vi "Associated Power Technologies 8500 Series Manual Mode.vi"() -> ()   [LabVIEW 2014]
doc: "This VI is an example for controlling the power source, APT-8500 series, of Associated Power Technologies. \n\nThe manual mode is a fundamental function to output a configured voltage ."
uses:
  <instrlib>/Associated Power Technologies 8500 Series/Public/Configure/Manual Mode/Manual Mode - Add File.vi
  <instrlib>/Associated Power Technologies 8500 Series/Public/Configure/Manual Mode/Manual Mode - Edit File.vi
  <instrlib>/Associated Power Technologies 8500 Series/Public/Configure/Manual Mode/Manual Mode - Configure Output Couple.vi
  <instrlib>/Associated Power Technologies 8500 Series/Public/Configure/Manual Mode/Manual Mode - Configure Range.vi
  <instrlib>/Associated Power Technologies 8500 Series/Public/Configure/Manual Mode/Manual Mode - Configure Output Waveform.vi
  <instrlib>/Associated Power Technologies 8500 Series/Public/Configure/Manual Mode/Manual Mode - Configure AC Voltage.vi
  <instrlib>/Associated Power Technologies 8500 Series/Public/Configure/Manual Mode/Manual Mode - Configure Frequency.vi
  <instrlib>/Associated Power Technologies 8500 Series/Public/Configure/Manual Mode/Manual Mode - Configure Start Angle.vi
  <instrlib>/Associated Power Technologies 8500 Series/Public/Configure/Manual Mode/Manual Mode - Configure DC Voltage.vi
  <instrlib>/Associated Power Technologies 8500 Series/Public/Configure/Manual Mode/Manual Mode - Configure Ramp up time.vi
  <instrlib>/Associated Power Technologies 8500 Series/Public/Configure/Manual Mode/Manual Mode - Configure High Limitation of Current.vi
  <instrlib>/Associated Power Technologies 8500 Series/Public/Configure/Manual Mode/Manual Mode - Configure High Limitation of Power.vi
  <instrlib>/Associated Power Technologies 8500 Series/Public/Configure/Manual Mode/Manual Mode - Configure Delay Time of High Limitation.vi
  <instrlib>/Associated Power Technologies 8500 Series/Public/Configure/Manual Mode/Manual Mode - Configure THD.vi
  <instrlib>/Associated Power Technologies 8500 Series/Public/Configure/Manual Mode/Manual Mode - Load File.vi
  <instrlib>/Associated Power Technologies 8500 Series/Public/Data/Measurement/Read All Measurements.vi
  <instrlib>/Associated Power Technologies 8500 Series/Associated Power Technologies 8500 Series.lvlib
panel:
  out "All Measurements":T1
  in  "File Name":string="EXAMPLE"
  in  "Stop":bool
  in  "Manual Mode Parameters":T2={"Couple"=2, "Waveform Type"=0, "Range"=0, "AC Voltage"=100.0, "DC Voltage"=0.0, "Frequency"=60.0, "Ramp Up Time(s)"=0.0, "Start Angle(degree)"=0, "A-HI(A)"=0.0, "P-HI(W)"=0, "Delay(s)"=0.0, "THD"=0.0} {"THD" min=0.0 max=46.0 step=0.1; "Couple" items=["AC", "DC", "ACDC"]; "Waveform Type" items=["Sine", "Triangle", "Square", "Clipped"]; "Range" items=["AUTO", "HIGH", "LOW"]; "AC Voltage" min=0.0 max=310.0; "DC Voltage" min=0.0 max=420.0; "Frequency" min=5.0 max=1200.0; "Ramp Up Time(s)" min=0.0 max=999.9 step=0.1; "Start Angle(degree)" max=359; "A-HI(A)" min=0.0; "Delay(s)" min=0.0 max=999.9 step=0.1}
  in  "Serial Configuration":T3={"Baud Rate"=115200, "Parity"=0, "Data Bits"=8, "Stop Bits"=10, "Flow Control"=0} {"Flow Control" items=["None", "XON/XOFF", "RTS/CTS", "XON/XOFF & RTS/CTS", "DTR/DSR", "XON/XOFF & DTR/DSR"]; "Stop Bits" items=["1.0"=10, "1.5"=15, "2.0"=20]; "Data Bits" items=["7"=7, "8"=8]; "Parity" items=["None", "Odd", "Even", "Mark", "Space"]; "Baud Rate" items=["300"=300, "600"=600, "1200"=1200, "2400"=2400, "4800"=4800, "9600"=9600, "19200"=19200, "38400"=38400, "115200"=115200]}
  in  "VISA resource name":refnum<visa-resource-name>
  # "Manual Mode Operation of APT-8500 Series"
  # "Initialization"
  # "Configurations"
  # "Meters"
  # "(c) 2020 Associated Power Technologies.  ALL RIGHTS RESERVED."
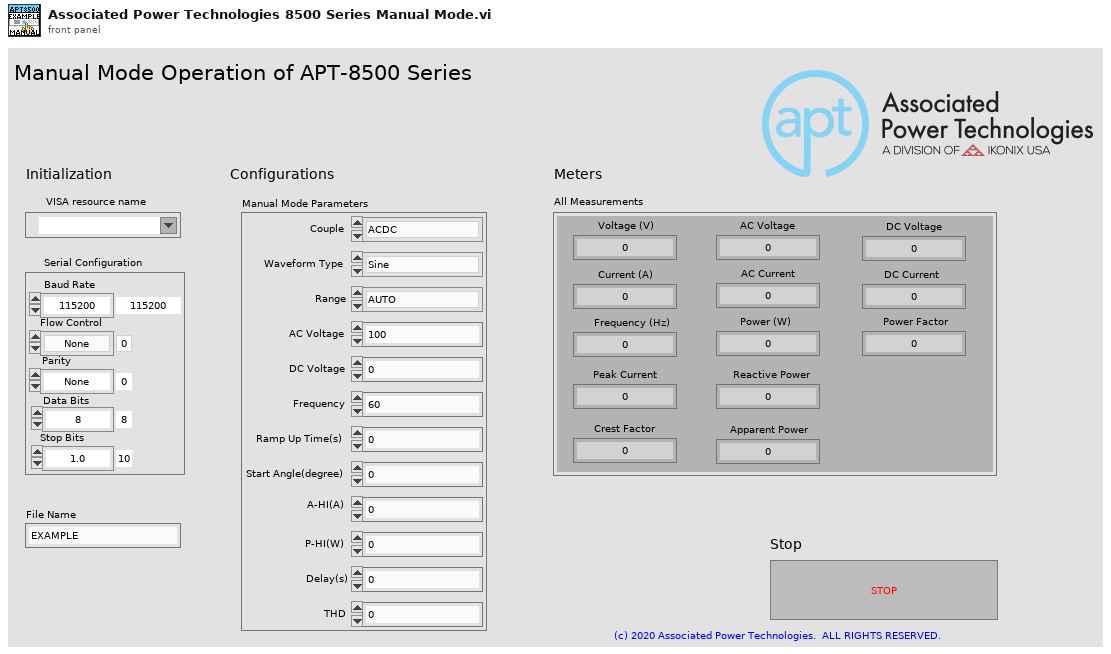
[diagram p1: front panel]
types:
  T1 = cluster{"Voltage (V)":dbl, "AC Voltage":dbl, "DC Voltage":dbl, "Current (A)":dbl, "AC Current":dbl, "DC Current":dbl, "Frequency (Hz)":dbl, "Power (W)":dbl, "Power Factor":dbl, "Peak Current":dbl, "Reactive Power":dbl, "Crest Factor":dbl, "Apparent Power":dbl}
  T2 = cluster{"Couple":u16, "Waveform Type":u16, "Range":u16, "AC Voltage":dbl, "DC Voltage":dbl, "Frequency":dbl, "Ramp Up Time(s)":dbl, "Start Angle(degree)":u16, "A-HI(A)":dbl, "P-HI(W)":u32, "Delay(s)":dbl, "THD":dbl}
  T3 = cluster{"Baud Rate":u32, "Parity":u16, "Data Bits":u16, "Stop Bits":u16, "Flow Control":u16}
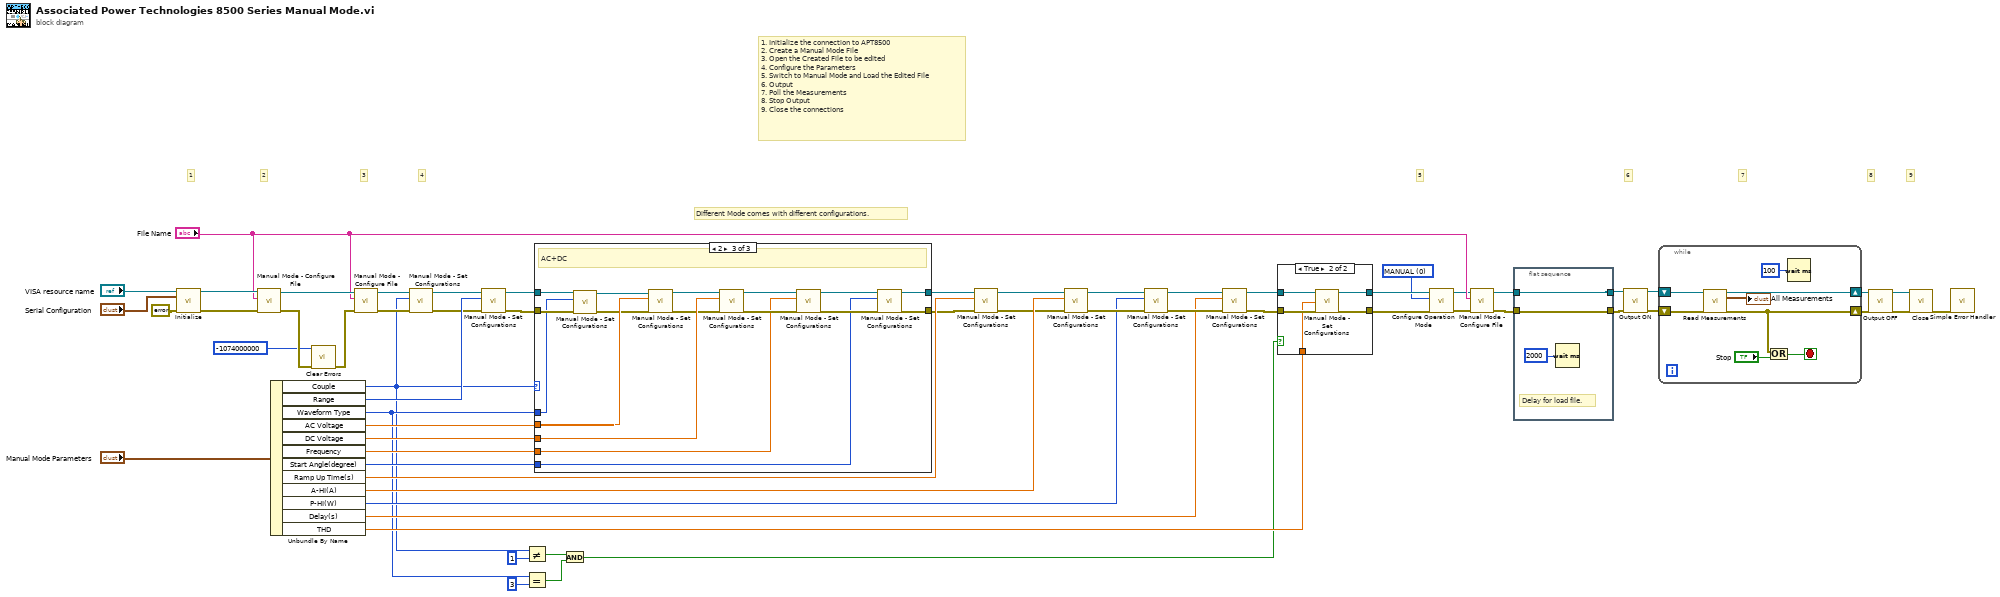
[diagram p0: block diagram]
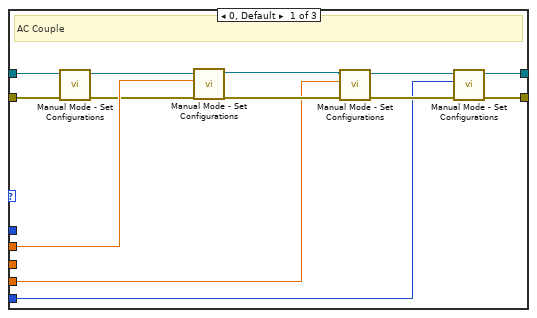
[diagram p3: hidden frame]
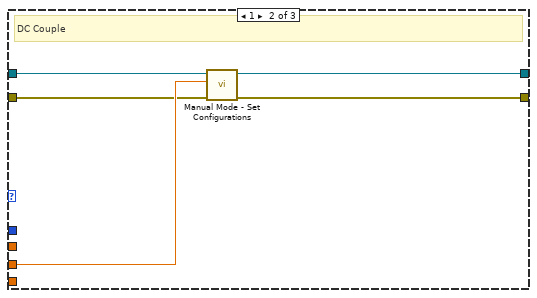
[diagram p4: hidden frame]
diagram:
  w3 = u16 0 items=["MANUAL", "LIST", "PULSE", "STEP"] ("Operation Mode")
  # "Different Mode comes with different configurations."
  # "1. Initialize the connection to APT8500\n2. Create a Manual Mode File\n3. Open the Created File to be edited\n4. Configure the Parameters\n5. Switch to Manual Mode and Load the Edited File\n6. Output\n7. Poll the Measurements\n8. Stop Output\n9. Close the connections"
  # "9"
  # "8"
  # "7"
  # "6"
  # "5"
  # "4"
  # "3"
  # "2"
  # "1"
  n1 = call <instrlib>:"Initialize.vi"("VISA resource name"="VISA resource name", "Serial Configuration"="Serial Configuration", "error in (no error)"=errorcluster {"status"=FALSE, "code"=0, "source"=""}) -> ("VISA resource name out"=w56:refnum<visa-resource-name>, "error out"=w57:errorcluster)  [unwired: 11 in]
  n2 = call-poly <instrlib>:"Manual Mode - Configure File.vi"("error in (no error)"=w57, "File Name"="File Name", "VISA resource name"=w56) -> ("error out"=w11:errorcluster, "VISA resource name out"=w55:refnum<visa-resource-name>)  [unwired: 7 in]
  n3 = Unbundle By Name("Manual Mode Parameters") -> ("Couple"=w26:u16, "Range"=w29:u16, "Waveform Type"=w28:u16, "AC Voltage"=w50:dbl, "DC Voltage"=w47:dbl, "Frequency"=w36:dbl, "Start Angle(degree)"=w32:u16, "Ramp Up Time(s)"=w33:dbl, "A-HI(A)"=w46:dbl, "P-HI(W)"=w43:u32, "Delay(s)"=w40:dbl, "THD"=w37:dbl)
  n4 = call <vilib>:"Clear Errors.vi"("error in (no error)"=w11, "specific error code to clear (0: all)"=-1074000000) -> ("error out"=w10:errorcluster)  [unwired: 4 in, 1 out]
  n5 = call-poly <instrlib>:"Manual Mode - Configure File.vi"("error in (no error)"=w10, "File Name"="File Name", "VISA resource name"=w55) -> ("error out"=w53:errorcluster, "VISA resource name out"=w54:refnum<visa-resource-name>)  [unwired: 7 in]
  n6 = call-poly <instrlib>:"Manual Mode - Set Configurations.vi"("error in (no error)"=w53, "Couple (AC)"=w26, "VISA resource name"=w54) -> ("error out"=w1:errorcluster, "VISA resource name out"=w2:refnum<visa-resource-name>)  [unwired: 7 in]
  n7 = call-poly <instrlib>:"Manual Mode - Set Configurations.vi"("error in (no error)"=w1, "Range (Auto)"=w29, "VISA resource name"=w2) -> ("error out"=w48:errorcluster, "VISA resource name out"=w49:refnum<visa-resource-name>)  [unwired: 7 in]
  n8 = Not Equal?(x=w26, y=u16 1) -> (x != y?=w23:bool)
  n9 = Equal?(x=w28, y=u16 3 ("x")) -> (x = y?=w24:bool)
  n10 = case shown="2" w26 {
    tunnel: w50 -> [w73 _ w95]
    tunnel: w49 -> [w64 w75 w83]
    tunnel: w48 -> [w62 w74 w81]
    tunnel: w47 -> [_ w78 w94]
    tunnel: [w66 w77 w86] -> w31
    tunnel: [w67 w76 w85] -> w30
    tunnel: w36 -> [w70 _ w89]
    tunnel: w32 -> [w65 _ w84]
    tunnel: w28 -> [_ _ w79]
    frame 0, Default {
      # "AC Couple"
      n11 = call-poly <instrlib>:"Manual Mode - Set Configurations.vi"("error in (no error)"=w62, "VISA resource name"=w64) -> ("error out"=w61:errorcluster, "VISA resource name out"=w63:refnum<visa-resource-name>)  [unwired: 8 in]
      n12 = call-poly <instrlib>:"Manual Mode - Set Configurations.vi"("error in (no error)"=w61, "AC Voltage (0)"=w73, "VISA resource name"=w63) -> ("error out"=w71:errorcluster, "VISA resource name out"=w72:refnum<visa-resource-name>)  [unwired: 7 in]
      n13 = call-poly <instrlib>:"Manual Mode - Set Configurations.vi"("error in (no error)"=w71, "Frequency (60)"=w70, "VISA resource name"=w72) -> ("error out"=w68:errorcluster, "VISA resource name out"=w69:refnum<visa-resource-name>)  [unwired: 7 in]
      n14 = call-poly <instrlib>:"Manual Mode - Set Configurations.vi"("error in (no error)"=w68, "Start Angle (0)"=w65, "VISA resource name"=w69) -> ("error out"=w67:errorcluster, "VISA resource name out"=w66:refnum<visa-resource-name>)  [unwired: 7 in]
    }
    frame 1 {
      # "DC Couple"
      n15 = call-poly <instrlib>:"Manual Mode - Set Configurations.vi"("error in (no error)"=w74, "DC Voltage (0)"=w78, "VISA resource name"=w75) -> ("error out"=w76:errorcluster, "VISA resource name out"=w77:refnum<visa-resource-name>)  [unwired: 7 in]
    }
    frame 2 {
      # "AC+DC"
      n16 = call-poly <instrlib>:"Manual Mode - Set Configurations.vi"("error in (no error)"=w81, "Waveform Type (Sine)"=w79, "VISA resource name"=w83) -> ("error out"=w80:errorcluster, "VISA resource name out"=w82:refnum<visa-resource-name>)  [unwired: 7 in]
      n17 = call-poly <instrlib>:"Manual Mode - Set Configurations.vi"("error in (no error)"=w80, "AC Voltage (0)"=w95, "VISA resource name"=w82) -> ("error out"=w92:errorcluster, "VISA resource name out"=w93:refnum<visa-resource-name>)  [unwired: 7 in]
      n18 = call-poly <instrlib>:"Manual Mode - Set Configurations.vi"("error in (no error)"=w92, "DC Voltage (0)"=w94, "VISA resource name"=w93) -> ("error out"=w91:errorcluster, "VISA resource name out"=w90:refnum<visa-resource-name>)  [unwired: 7 in]
      n19 = call-poly <instrlib>:"Manual Mode - Set Configurations.vi"("error in (no error)"=w91, "Frequency (60)"=w89, "VISA resource name"=w90) -> ("error out"=w88:errorcluster, "VISA resource name out"=w87:refnum<visa-resource-name>)  [unwired: 7 in]
      n20 = call-poly <instrlib>:"Manual Mode - Set Configurations.vi"("error in (no error)"=w88, "Start Angle (0)"=w84, "VISA resource name"=w87) -> ("error out"=w85:errorcluster, "VISA resource name out"=w86:refnum<visa-resource-name>)  [unwired: 7 in]
    }
  }
  n21 = And(x=w23, y=w24) -> (x .and. y?=w22:bool)
  n22 = call-poly <instrlib>:"Manual Mode - Set Configurations.vi"("error in (no error)"=w30, "Ramp Up Time (0)"=w33, "VISA resource name"=w31) -> ("error out"=w34:errorcluster, "VISA resource name out"=w35:refnum<visa-resource-name>)  [unwired: 7 in]
  n23 = call-poly <instrlib>:"Manual Mode - Set Configurations.vi"("error in (no error)"=w34, "A-HI(0)"=w46, "VISA resource name"=w35) -> ("error out"=w44:errorcluster, "VISA resource name out"=w45:refnum<visa-resource-name>)  [unwired: 7 in]
  n24 = call-poly <instrlib>:"Manual Mode - Set Configurations.vi"("error in (no error)"=w44, "P-HI(0)"=w43, "VISA resource name"=w45) -> ("error out"=w41:errorcluster, "VISA resource name out"=w42:refnum<visa-resource-name>)  [unwired: 7 in]
  n25 = call-poly <instrlib>:"Manual Mode - Set Configurations.vi"("error in (no error)"=w41, "Delay(0)"=w40, "VISA resource name"=w42) -> ("error out"=w38:errorcluster, "VISA resource name out"=w39:refnum<visa-resource-name>)  [unwired: 7 in]
  n26 = case shown="True" w22 {
    tunnel: w39 -> [w97 w102]
    tunnel: w38 -> [w96 w101]
    tunnel: w37 -> [_ w100]
    tunnel: [w97 w99] -> w6
    tunnel: [w96 w98] -> w5
    frame False {
    }
    frame True {
      n27 = call-poly <instrlib>:"Manual Mode - Set Configurations.vi"("error in (no error)"=w101, "THD (0)"=w100, "VISA resource name"=w102) -> ("error out"=w98:errorcluster, "VISA resource name out"=w99:refnum<visa-resource-name>)  [unwired: 7 in]
    }
  }
  n28 = call <instrlib>:"Configure Operation Mode.vi"("error in (no error)"=w5, "Operation Mode (MANUAL)"=w3, "VISA resource name"=w6) -> ("error out"=w4:errorcluster, "VISA resource name out"=w7:refnum<visa-resource-name>)  [unwired: 7 in]
  n29 = call-poly <instrlib>:"Manual Mode - Configure File.vi"("error in (no error)"=w4, "File Name"="File Name", "VISA resource name"=w7) -> ("error out"=w12:errorcluster, "VISA resource name out"=w14:refnum<visa-resource-name>)  [unwired: 7 in]
  n30 = flat-sequence {
    tunnel: [w105] -> w15
    tunnel: w14 -> [w105]
    tunnel: [w104] -> w13
    tunnel: w12 -> [w104]
    frame #0 {
      # "Delay for load file."
      n31 = Wait (ms)(milliseconds to wait=u32 2000) -> ()  [unwired: 1 out]
    }
  }
  n32 = call <instrlib>:"Output ON.vi"("VISA resource name"=w15, "error in (no error)"=w13) -> ("VISA resource name out"=w21:refnum<visa-resource-name>, "error out"=w20:errorcluster)  [unwired: 12 in]
  n33 = while {
    shift-right: [w107] -> w18
    shift-left: w21 -> [w110]
    shift-right: [w108] -> w19
    shift-left: w20 -> [w109]
    stop <- w113 stop-if-true
    n34 = call-poly <instrlib>:"Read Measurements.vi"("VISA resource name"=w110, "error in (no error)"=w109) -> ("VISA resource name out"=w107:refnum<visa-resource-name>, "All Measurements"=→"All Measurements":T1, "error out"=w108:errorcluster)  [unwired: 11 in]
    n35 = Or(x=w108, y="Stop") -> (x .or. y?=w113:bool)
    n36 = Wait (ms)(milliseconds to wait=u32 100) -> ()  [unwired: 1 out]
  }
  n37 = call <instrlib>:"Output OFF.vi"("VISA resource name"=w18, "error in (no error)"=w19) -> ("VISA resource name out"=w17:refnum<visa-resource-name>, "error out"=w16:errorcluster)  [unwired: 12 in]
  n38 = call <instrlib>:"Close.vi"("VISA resource name"=w17, "error in (no error)"=w16) -> ("error out"=w8:errorcluster)  [unwired: 13 in]
  n39 = call <vilib>:"Simple Error Handler.vi"("error in (no error)"=w8) -> ()  [unwired: 4 in, 5 out]
